vi "Reset ACK.vi"(8 "error in (no error)":errorcluster, 11 "MotionComm in":refnum<class "MotionComm.lvclass">) -> (0 "error out":errorcluster, 3 "MotionComm out":refnum<class "MotionComm.lvclass">)   [LabVIEW 2018, in "MotionComm.lvclass"]
doc: "at the beginning of a move that needs to be acked\nreset the ACK channel by flushing the ACK comm que."
uses:
  MotionComm.lvclass
  MotionComm.lvclass/MotionComm.ctl
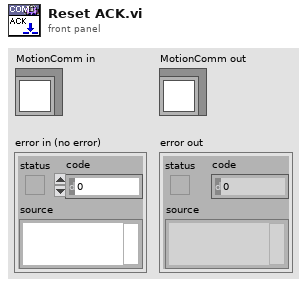
[diagram p1: front panel]
types:
  T1 = typedef "MessageQue.lvlib/MessageQue.ctl" = refnum<queue>
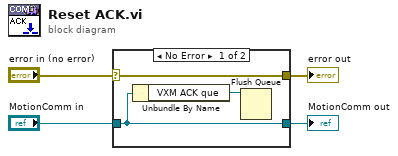
[diagram p0: block diagram]
diagram:
  n1 = case shown="No Error" "error in (no error)" {
    selector: "error in (no error)" -> [w7 w9]
    tunnel: [w7 w9] -> w3
    tunnel: [w6 w8] -> w1
    tunnel: "MotionComm in" -> [w6 w8]
    frame No Error {
      n2 = Unbundle By Name(w6) -> ("VXM ACK que"=w5:T1)
      n3 = Flush Queue(queue=w5) -> ()  [unwired: 1 in, 3 out]
    }
    frame Error {
    }
  }
  "error out" <- w3
  "MotionComm out" <- w1
